vi "SigSyn (G3)-Compute Max Level (wrapper).vi"(0 "Stimulus Channel":T1={"Waveform"={"Type"=enum."OFF", "Tone"={"Frequency (kHz)"=0.0, "Phase (cycles)"=0.0, "Random phase"=FALSE}, "Pulse Train"={"Pulse width (us)"=0.0, "Pulse rate (Hz)"=0.0, "Gap (ms)"=0.0, "Polarity"=enum."POS", "PT State"={"Template"=[], "Nperiod"=0, "Index"=0, "Pulse Rate (Hz)"=0.0, "Phase (cycles)"=0.0, "Noff"=0}, "Asynch"=FALSE}, "Noise"={"Properties"={"InvFilt"=FALSE, "Aweight"=FALSE, "Seed"=0, "Tokens"=0, "Brickwall"=FALSE}, "Data"={"TokenNum"=0}}, "File"={"Filename"=path "", "Signal"=[], "Channel"=0, "stream"=FALSE, "offset"=0, "nreps"=0, "loops"=0, "Randomize"=FALSE, "order"=[], "Seed"=0, "Tokens"=0}, "FMSweep"={"Rate (oct/s)"=0.0, "Fmin (Hz)"=0.0, "Fmax (Hz)"=0.0, "Ramp (ms)"=0.0, "Linear"=FALSE}, "Chirp Train"={"Params"={"Fmin (kHz)"=4.0, "Fmax (kHz)"=64.0, "Compensate"=FALSE, "Duration (ms)"=2.0}, "Data"={"WF"=[]}}, "Complex Tone"={"Params"={"F0 (Hz)"=0.0, "Band"={"Flow (Hz)"=0.0, "Fhigh (Hz)"=0.0}, "Phase"=enum."Cosine", "Min F0 (Hz)"=0.0, "Max F0 (Hz)"=0.0, "ContinRandPhase"=FALSE, "Max peak factor"=inf, "Max mod depth"=2.0, "MinHarmNum"=0, "MaxHarmNum"=0, "Level Mode"=enum."per component", "% jitter"=0.0}, "Data"={"Ncomp"=0, "MinHarm"=0, "Phase"=[], "Amplitude"=[], "Npts/frame"=0, "Last F0"=0.0, "Fmin"=0.0, "Fmax"=0.0, "Lslope"=0.0, "randphase"=FALSE, "overall rms"=FALSE, "fmult"=[], "jittered"=FALSE}}, "FM"={"Carrier (kHz)"=0.0, "ModRate (Hz)"=0.0, "Depth (Hz)"=0.0, "Phase (cycles)"=0.0}, "Vowel"={"Freqs"="", "Set level"=enum."Total", "Freq"=[], "weights"=[]}, "Ramp"={"Duration (ms)"=0.0}}, "Filter"={"Type"=enum."Lowpass", "CF (kHz)"=0.0, "BW (kHz)"=0.0, "Cascade"=FALSE, "Quadrature"=FALSE, "Scale Factor"=0.0, "Stages"=[], "Class"=enum."Elliptic", "Order"=0, "BWUnits"=enum."Linear"}, "Burst"={"Active"=FALSE, "Delay (ms)"=0.0, "Duration (ms)"=0.0, "Ramp (ms)"=0.0, "Rate (Hz)"=0.0, "Trepeat (ms)"=0.0, "Repeat"=FALSE}, "Level"={"Level"=0.0, "Units"=enum."dB atten", "Max"=0.0, "Data"={"Multiplier"=0.0, "Cal File"=path "", "Cal"={"Freq (Hz)"=[], "Mag (dB SPL)"=[], "Phase (deg)"=[]}, "audiogram"=path ""}}, "Name"="", "Advanced"={"AltPol"=FALSE, "Var"="", "Expr"=""}, "SAM"={"Active"=FALSE, "Frequency (Hz)"=0.0, "Depth"=0.0, "Init Phase (cycles)"=0.0, "phase (degrees)"=0.0, "Asynch"=FALSE}, "Destination"={"Name"="", "Num"=0}} {"Filter"."Stages"."IIR Filter"."Forward Coefficients" format="%.4f"; "Filter"."Stages"."IIR Filter"."Reverse Coefficients" format="%.4f"}, 7 "Sampling Rate (Hz)":dbl, 9 "Npts":i32, 11 "error in (no error)":errorcluster) -> (4 "Stimulus Channel out":T1={"Waveform"={"Type"=enum."OFF", "Tone"={"Frequency (kHz)"=0.0, "Phase (cycles)"=0.0, "Random phase"=FALSE}, "Pulse Train"={"Pulse width (us)"=0.0, "Pulse rate (Hz)"=0.0, "Gap (ms)"=0.0, "Polarity"=enum."POS", "PT State"={"Template"=[], "Nperiod"=0, "Index"=0, "Pulse Rate (Hz)"=0.0, "Phase (cycles)"=0.0, "Noff"=0}, "Asynch"=FALSE}, "Noise"={"Properties"={"InvFilt"=FALSE, "Aweight"=FALSE, "Seed"=0, "Tokens"=0, "Brickwall"=FALSE}, "Data"={"TokenNum"=0}}, "File"={"Filename"=path "", "Signal"=[], "Channel"=0, "stream"=FALSE, "offset"=0, "nreps"=0, "loops"=0, "Randomize"=FALSE, "order"=[], "Seed"=0, "Tokens"=0}, "FMSweep"={"Rate (oct/s)"=0.0, "Fmin (Hz)"=0.0, "Fmax (Hz)"=0.0, "Ramp (ms)"=0.0, "Linear"=FALSE}, "Chirp Train"={"Params"={"Fmin (kHz)"=4.0, "Fmax (kHz)"=64.0, "Compensate"=FALSE, "Duration (ms)"=2.0}, "Data"={"WF"=[]}}, "Complex Tone"={"Params"={"F0 (Hz)"=0.0, "Band"={"Flow (Hz)"=0.0, "Fhigh (Hz)"=0.0}, "Phase"=enum."Cosine", "Min F0 (Hz)"=0.0, "Max F0 (Hz)"=0.0, "ContinRandPhase"=FALSE, "Max peak factor"=inf, "Max mod depth"=2.0, "MinHarmNum"=0, "MaxHarmNum"=0, "Level Mode"=enum."per component", "% jitter"=0.0}, "Data"={"Ncomp"=0, "MinHarm"=0, "Phase"=[], "Amplitude"=[], "Npts/frame"=0, "Last F0"=0.0, "Fmin"=0.0, "Fmax"=0.0, "Lslope"=0.0, "randphase"=FALSE, "overall rms"=FALSE, "fmult"=[], "jittered"=FALSE}}, "FM"={"Carrier (kHz)"=0.0, "ModRate (Hz)"=0.0, "Depth (Hz)"=0.0, "Phase (cycles)"=0.0}, "Vowel"={"Freqs"="", "Set level"=enum."Total", "Freq"=[], "weights"=[]}, "Ramp"={"Duration (ms)"=0.0}}, "Filter"={"Type"=enum."Lowpass", "CF (kHz)"=0.0, "BW (kHz)"=0.0, "Cascade"=FALSE, "Quadrature"=FALSE, "Scale Factor"=0.0, "Stages"=[], "Class"=enum."Elliptic", "Order"=0, "BWUnits"=enum."Linear"}, "Burst"={"Active"=FALSE, "Delay (ms)"=0.0, "Duration (ms)"=0.0, "Ramp (ms)"=0.0, "Rate (Hz)"=0.0, "Trepeat (ms)"=0.0, "Repeat"=FALSE}, "Level"={"Level"=0.0, "Units"=enum."dB atten", "Max"=0.0, "Data"={"Multiplier"=0.0, "Cal File"=path "", "Cal"={"Freq (Hz)"=[], "Mag (dB SPL)"=[], "Phase (deg)"=[]}, "audiogram"=path ""}}, "Name"="", "Advanced"={"AltPol"=FALSE, "Var"="", "Expr"=""}, "SAM"={"Active"=FALSE, "Frequency (Hz)"=0.0, "Depth"=0.0, "Init Phase (cycles)"=0.0, "phase (degrees)"=0.0, "Asynch"=FALSE}, "Destination"={"Name"="", "Num"=0}} {"Filter"."Stages"."IIR Filter"."Forward Coefficients" format="%.4f"; "Filter"."Stages"."IIR Filter"."Reverse Coefficients" format="%.4f"}, 14 "Max Level":dbl, 15 "error out":errorcluster)   [LabVIEW 2020]
uses:
  XControls/Stimulus Channel (G3)/Full Stimulus Channel Data.ctl
  XControls/Waveform XControls/Waveform (G3)/Waveform Data.ctl
  Waveform VIs/Waveform Enum (V3).ctl
  XControls/Waveform XControls/Tone (G3)/Tone.Properties.ctl
  Waveform VIs/Pulse Train VIs/Pulse Train Params.ctl
  Waveform VIs/Pulse Train VIs/Pulse Polarity.ctl
  Waveform VIs/Pulse Train VIs/PT-Continuous State.ctl
  Waveform VIs/Noise VIs/Noise (G3).ctl
  Waveform VIs/Noise VIs/Noise (G3).Properties.ctl
  Waveform VIs/Noise VIs/Noise (G3).Data.ctl
  Waveform VIs/File VIs/StimFile-Params.ctl
  Waveform VIs/FM Sweep VIs/FM Sweep Params.ctl
  Waveform VIs/Chirp Train VIs/Chirp Train.ctl
  Waveform VIs/Chirp Train VIs/Chirp Train Params.ctl
  Waveform VIs/Complex Tone VIs/CT-Params.ctl
  Waveform VIs/Complex Tone VIs/CT-Phase Enum.ctl
  Waveform VIs/Complex Tone VIs/CT-Runtime Data.ctl
  XControls/Waveform XControls/FM Tone/Data.ctl
  XControls/Waveform XControls/Vowel/Vowel.Properties.ctl
  Waveform VIs/Ramp VIs/Ramp.Properties.ctl
  XControls/Filter (G3)/Filter Data.ctl
  XControls/Filter (G3)/Filter Type.ctl
  Filter VIs/Filter-Bandwidth Units.ctl
  Controls/Burst XCtl/Burst Data.ctl
  XControls/Level (G3)/Level Data.ctl
  XControls/Level (G3)/Level Units (G3).ctl
  XControls/Advanced Options (G3)/Advanced Options (G3).ctl
  Modulation VIs/SAM VIs/SAM Params.ctl
  Typedefs/Destination.ctl
  Controls/Burst XCtl/Burst Control.xctl
  XControls/Level (G3)/Level (G3).xctl
  XControls/Waveform XControls/Waveform (G3)/Waveform (G3).xctl
  XControls/Stimulus Channel (G3)/Stimulus Channel (G3).xctl
  XControls/Filter (G3)/Filter (G3).xctl
  XControls/Advanced Options (G3)/Advanced Options (G3).xctl
  XControls/Waveform XControls/Tone (G3)/Tone (G3).xctl
  XControls/Waveform XControls/FM Tone/FM Tone.xctl
  XControls/Waveform XControls/Vowel/Vowel.xctl
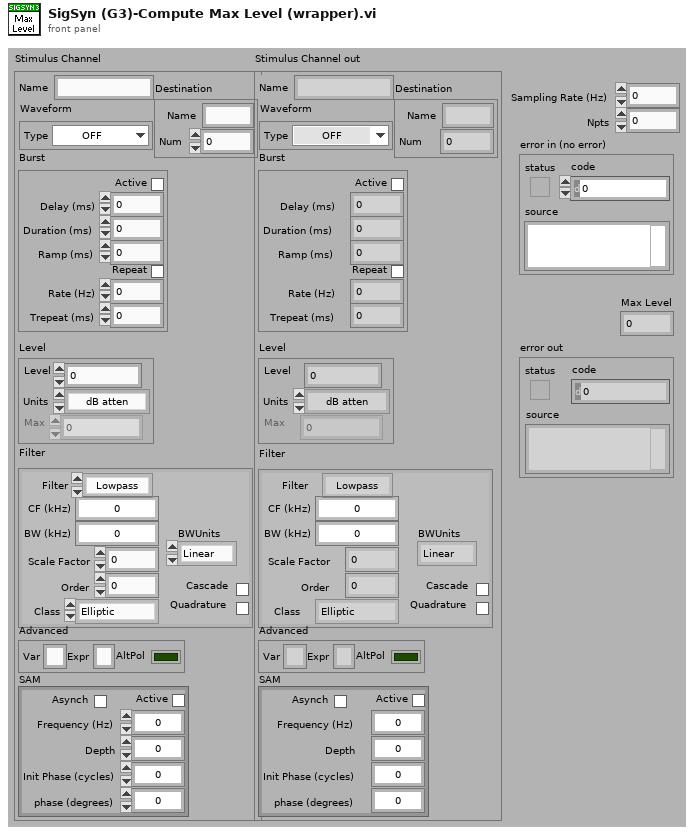
[diagram p1: front panel]
types:
  T1 = typedef "Stimulus Channel (G3).xctl/Full Stimulus Channel Data.ctl" = cluster{"Waveform":T2, "Filter":T21, "Burst":T24, "Level":T25, "Name":string, "Advanced":T27, "SAM":T28, "Destination":T29}
  T2 = typedef "Waveform (G3).xctl/Waveform Data.ctl" = cluster{"Type":T3, "Tone":T4, "Pulse Train":T5, "Noise":T8, "File":T11, "FMSweep":T12, "Chirp Train":T13, "Complex Tone":cluster{"Params":T15, "Data":T17}, "FM":T18, "Vowel":T19, "Ramp":T20}
  T3 = typedef "Waveform Enum (V3).ctl" = enum16{"OFF", "Tone", "Noise", "Pulse Train", "File", "FM Sweep", "Chirp Train", "Complex Tone", "FM Tone", "Vowel", "Ramp"}
  T4 = typedef "Tone (G3).xctl/Tone.Properties.ctl" = cluster{"Frequency (kHz)":dbl, "Phase (cycles)":dbl, "Random phase":bool}
  T5 = typedef "Pulse Train Params.ctl" = cluster{"Pulse width (us)":dbl, "Pulse rate (Hz)":dbl, "Gap (ms)":dbl, "Polarity":T6, "PT State":T7, "Asynch":bool}
  T6 = typedef "Pulse Polarity.ctl" = enum16{"POS", "NEG", "POS-NEG", "NEG-POS"}
  T7 = typedef "PT-Continuous State.ctl" = cluster{"Template":dbl[], "Nperiod":i32, "Index":i32, "Pulse Rate (Hz)":dbl, "Phase (cycles)":dbl, "Noff":i32}
  T8 = typedef "Noise (G3).ctl" = cluster{"Properties":T9, "Data":T10}
  T9 = typedef "Noise (G3).Properties.ctl" = cluster{"InvFilt":bool, "Aweight":bool, "Seed":i32, "Tokens":i32, "Brickwall":bool}
  T10 = typedef "Noise (G3).Data.ctl" = cluster{"TokenNum":i32}
  T11 = typedef "StimFile-Params.ctl" = cluster{"Filename":path, "Signal":dbl[], "Channel":i32, "stream":bool, "offset":i32, "nreps":i32, "loops":i32, "Randomize":bool, "order":i32[], "Seed":i32, "Tokens":i32}
  T12 = typedef "FM Sweep Params.ctl" = cluster{"Rate (oct/s)":dbl, "Fmin (Hz)":dbl, "Fmax (Hz)":dbl, "Ramp (ms)":dbl, "Linear":bool}
  T13 = typedef "Chirp Train.ctl" = cluster{"Params":T14, "Data":cluster{"WF":dbl[]}}
  T14 = typedef "Chirp Train Params.ctl" = cluster{"Fmin (kHz)":dbl, "Fmax (kHz)":dbl, "Compensate":bool, "Duration (ms)":dbl}
  T15 = typedef "CT-Params.ctl" = cluster{"F0 (Hz)":dbl, "Band":cluster{"Flow (Hz)":dbl, "Fhigh (Hz)":dbl}, "Phase":T16, "Min F0 (Hz)":dbl, "Max F0 (Hz)":dbl, "ContinRandPhase":bool, "Max peak factor":dbl, "Max mod depth":dbl, "MinHarmNum":i32, "MaxHarmNum":i32, "Level Mode":enum16{"per component", "overall rms"}, "% jitter":dbl}
  T16 = typedef "CT-Phase Enum.ctl" = enum16{"Cosine", "Random", "Alternating"}
  T17 = typedef "CT-Runtime Data.ctl" = cluster{"Ncomp":i32, "MinHarm":i32, "Phase":dbl[], "Amplitude":dbl[], "Npts/frame":i32, "Last F0":dbl, "Fmin":dbl, "Fmax":dbl, "Lslope":dbl, "randphase":bool, "overall rms":bool, "fmult":dbl[], "jittered":bool}
  T18 = typedef "FM Tone.xctl/Data.ctl" = cluster{"Carrier (kHz)":dbl, "ModRate (Hz)":dbl, "Depth (Hz)":dbl, "Phase (cycles)":dbl}
  T19 = typedef "Vowel.xctl/Vowel.Properties.ctl" = cluster{"Freqs":string, "Set level":enum16{"Total", "Per component"}, "Freq":dbl[], "weights":dbl[]}
  T20 = typedef "Ramp.Properties.ctl" = cluster{"Duration (ms)":dbl}
  T21 = typedef "Filter (G3).xctl/Filter Data.ctl" = cluster{"Type":T22, "CF (kHz)":dbl, "BW (kHz)":dbl, "Cascade":bool, "Quadrature":bool, "Scale Factor":dbl, "Stages":cluster{"IIR Filter":cluster{"filter structure":enum32{"IIR 2nd Order", "IIR 4th Order"}, "Reverse Coefficients":dbl[], "Forward Coefficients":dbl[]}, "State":dbl[]}[], "Class":enum16{"Elliptic", "Butterworth"}, "Order":i32, "BWUnits":T23}
  T22 = typedef "Filter (G3).xctl/Filter Type.ctl" = enum16{"OFF", "Lowpass", "Highpass", "Bandpass", "Bandstop"}
  T23 = typedef "Filter-Bandwidth Units.ctl" = enum16{"Linear", "Octaves", "Min-Max"}
  T24 = typedef "Burst Control.xctl/Burst Data.ctl" = cluster{"Active":bool, "Delay (ms)":dbl, "Duration (ms)":dbl, "Ramp (ms)":dbl, "Rate (Hz)":dbl, "Trepeat (ms)":dbl, "Repeat":bool}
  T25 = typedef "Level (G3).xctl/Level Data.ctl" = cluster{"Level":dbl, "Units":T26, "Max":dbl, "Data":cluster{"Multiplier":dbl, "Cal File":path, "Cal":cluster{"Freq (Hz)":dbl[], "Mag (dB SPL)":dbl[], "Phase (deg)":dbl[]}, "audiogram":path}}
  T26 = typedef "Level (G3).xctl/Level Units (G3).ctl" = enum16{"dB atten", "dB SPL", "dB re 1 Vrms", "dB V/Hz½", "mW", "dB HL", "Volts", "dB mW"}
  T27 = typedef "Advanced Options (G3).xctl/Advanced Options (G3).ctl" = cluster{"AltPol":bool, "Var":string, "Expr":string}
  T28 = typedef "SAM Params.ctl" = cluster{"Active":bool, "Frequency (Hz)":dbl, "Depth":dbl, "Init Phase (cycles)":dbl, "phase (degrees)":dbl, "Asynch":bool}
  T29 = typedef "Destination.ctl" = cluster{"Name":string, "Num":i32}
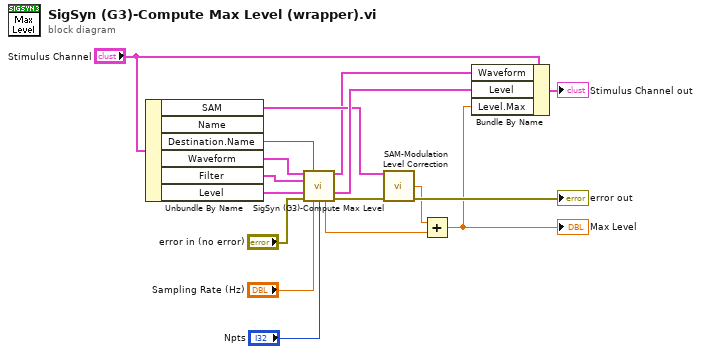
[diagram p0: block diagram]
diagram:
  n1 = Unbundle By Name("Stimulus Channel") -> ("SAM"=w5:T28, "Destination.Name"=w1:string, "Waveform"=w9:T2, "Filter"=w8:T21, "Level"=w17:T25)  [unwired: 1 out]
  n2 = call "SigSyn (G3)-Compute Max Level.vi"("Waveform In"=w9, "Destination"=w1, "Filter"=w8, "Level"=w17, "error in (no error)"="error in (no error)", "Sampling Rate (Hz)"="Sampling Rate (Hz)", "Npts"="Npts") -> ("Waveform Out"=w2:T2, "Level out"=w11:T25, "Max Level"=w13:dbl, "error out"=w7:errorcluster)  [unwired: 5 in]
  n3 = call "SAM-Modulation Level Correction.vi"("SAM"=w5, "error in (no error)"=w7) -> ("Correction (dB)"=w4:dbl, "error out"=→"error out":errorcluster)  [unwired: 12 in]
  n4 = Add(x=w4, y=w13) -> (x+y=w3:dbl)
  "Max Level" <- w3
  n5 = Bundle By Name(cluster="Stimulus Channel", "Waveform"=w2, "Level"=w11, "Level.Max"=w3) -> (→"Stimulus Channel out":T1)
